vi "Q14070-Z030装调整机构.vi"() -> ()   [LabVIEW 2013]
panel:
  out "error out 3":errorcluster
  out "型号数量":i32=10
  out "KSJJ":string
  out "FGCS":string
  out "03RFID":string
  out "RFID读取完成":bool
  out "RFID读取触发":bool
  out "芯片ID":string
  out "产品ID":string
  in  "锁紧螺母批次号":string
  in  "调整螺塞批次号":string
  in  "弹簧批次号":string
  in  "O型圈批次号":string
  in  "支撑座批次号":string
  in  "复位按钮":bool
  in  "员工权限":bool
  in  "停止":bool
  in  "联线按钮":bool
  out "通讯状态":bool
  in  "选项卡控件 2":enum32{"自动", "手动", "参数查询"}(tab)
  out "本序完成":bool
  out "本序合格":bool
  out "上序完成":bool
  out "上序合格":bool
  out "取料操作状态":string
  out "取料工步号":dbl
  out "涂脂操作状态":string
  out "涂脂工步号":dbl
  out "流水线操作状态":string
  in  "流水线工步号":dbl
  out "报警提示":string
  out "报警工步号":dbl
  out "I上工位在位":bool
  out "I本工位在位":bool
  out "I下工位在位":bool
  out "I旋转气缸原位  2":bool
  out "I顶升气缸下位 2":bool
  out "I顶升气缸上位  2":bool
  out "I旋转气缸进位 2":bool
  out "I胶瓶在位":bool
  out "I辅具在位":bool
  out "I横孔涂脂在位":bool
  in  "M支撑座手动涂脂有效":bool
  in  "M图像识别涂脂开":bool
  in  "M图像识别触发":bool
  in  "M本工位放行":bool
  in  "M流水线旋转气缸原位":bool
  in  "M上工位放行":bool
  in  "M流水线顶升气缸下降":bool
  in  "M流水线旋转气缸旋转":bool
  in  "M横孔涂脂开":bool
  in  "M流水线顶升气缸顶升":bool
  out "I下工位在位":bool
  out "I上工位在位":bool
  out "I本工位在位":bool
  out "I旋转气缸进位":bool
  out "I顶升气缸上位":bool
  out "I顶升气缸下位":bool
  out "I旋转气缸原位":bool
  in  "参数修改":bool
  in  "参数查询":bool
  in  "参数列表":string[][](table)
  in  "员工ID":string
  out "员工姓名":string
  in  "型号选择":u16(ring)=1 items=["J706", "J709"]
  in  "参数加载":bool
  out "Q场景切换启动2":bool
  out "Q场景切换启动1":bool
  out "备用取料":i16=4
  out "error out 2":errorcluster
  out "ADODB._Connection Out":refnum<k7>
  out "error out":errorcluster
  out "Q场景切换 4":bool
  out "Q场景切换 3":bool
  out "Q场景切换 2":bool
  out "Q场景切换":bool
  out "场景切换选择":i16=4
  out "横孔涂脂设定次数":i16=4
  out "齿条支撑座涂脂设定次数":i16=4
  in  "M备用取料":bool
  out "产品选型":dbl
  # "芜湖机械转向器装配线"
  # "Z030 装调整机构"
  # "湖北唯思凌科装备制造有限公司 设计开发 (C)2015"
  # "Q14070机械转向器装配线"
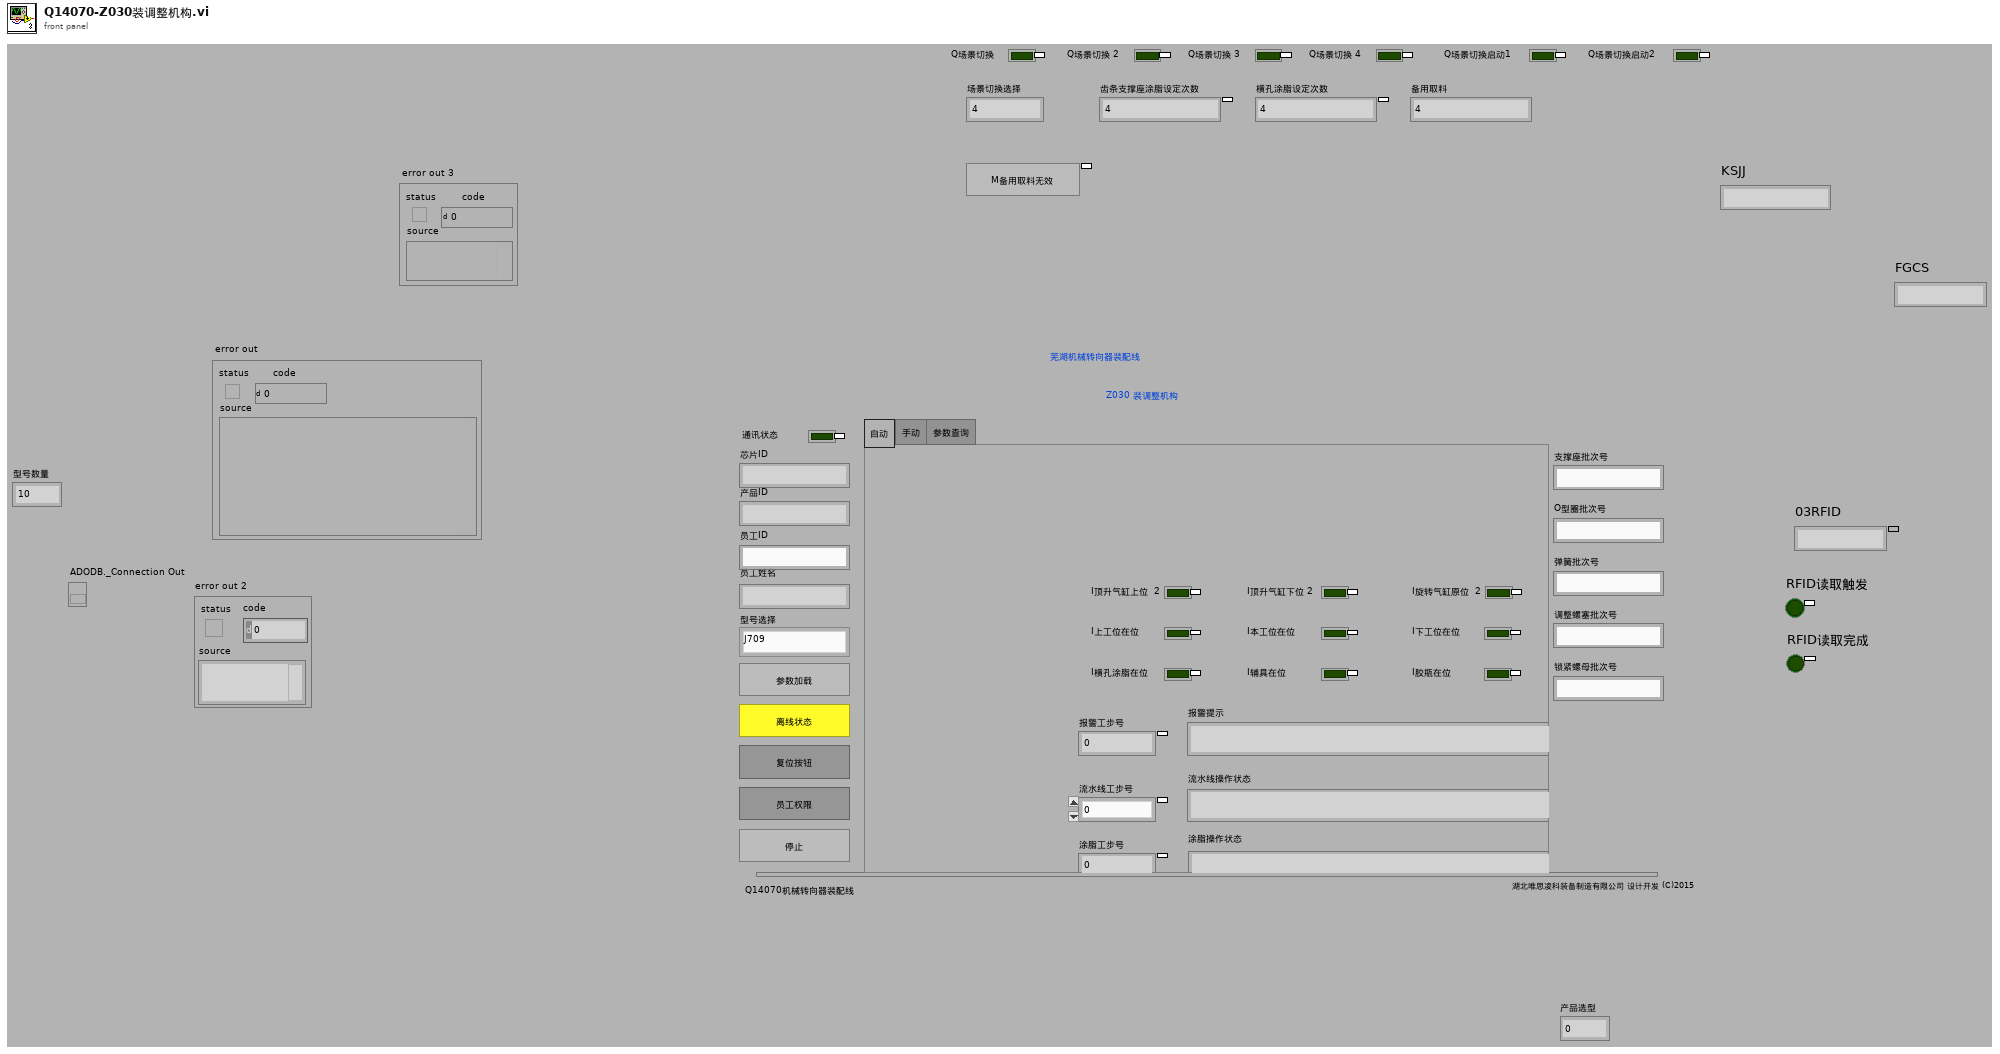
[diagram p1: front panel]
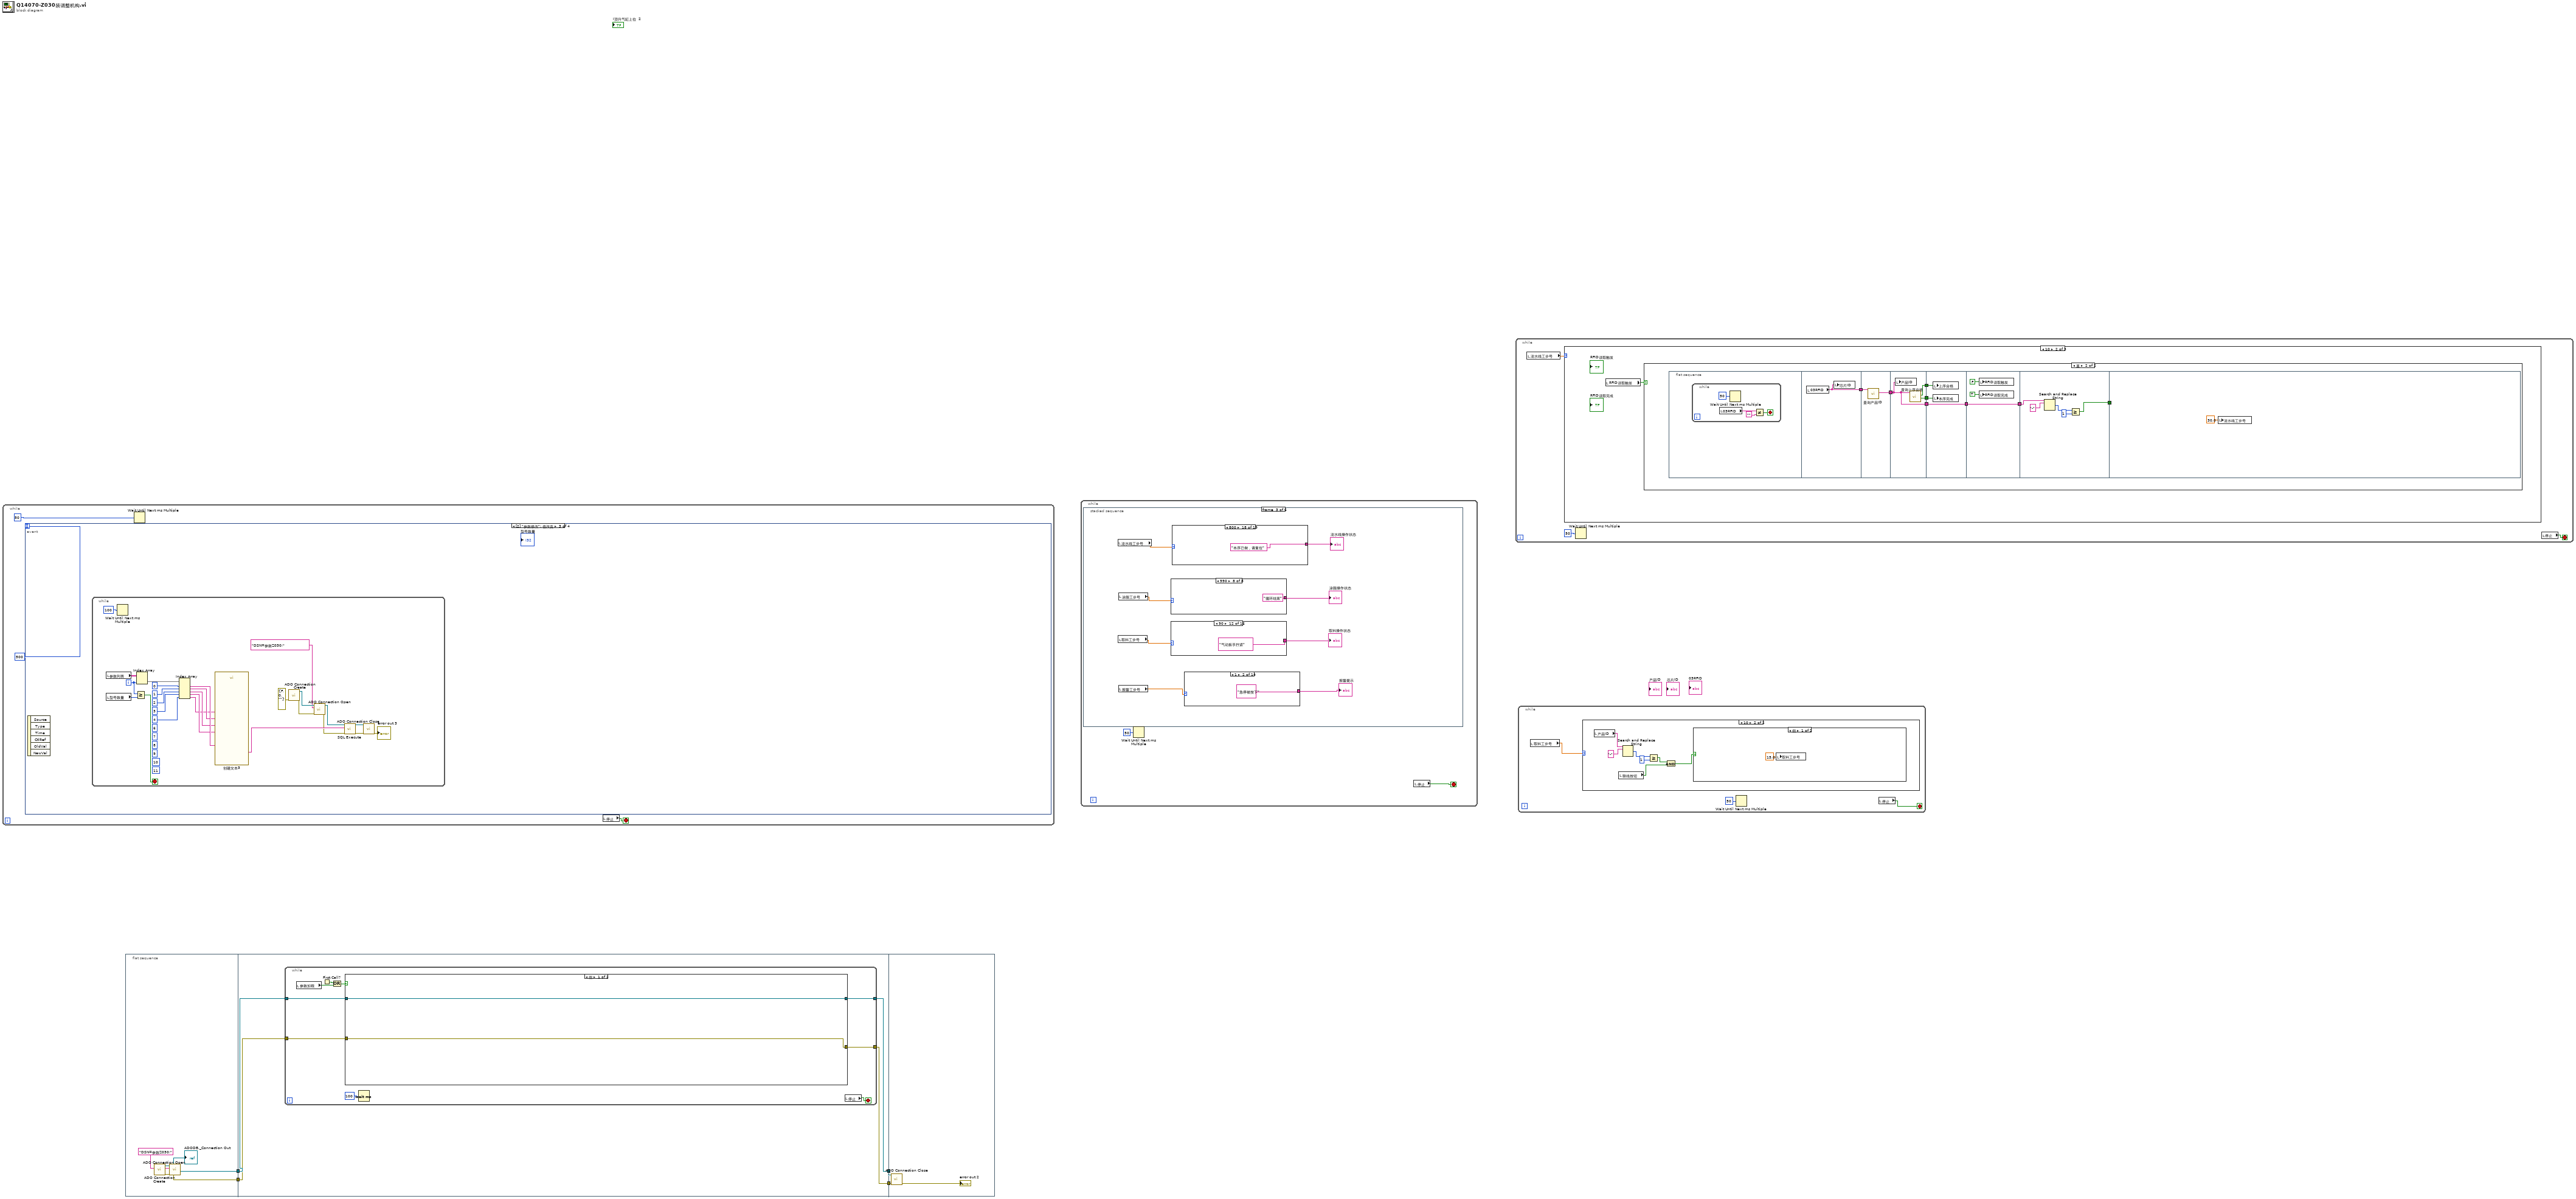
[diagram p0: block diagram]
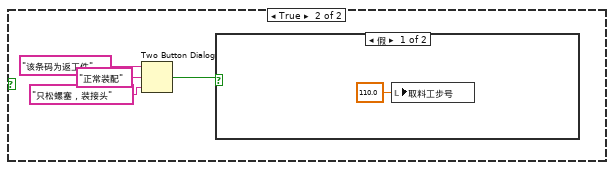
[diagram p3: hidden frame]
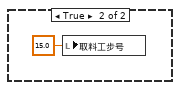
[diagram p4: hidden frame]
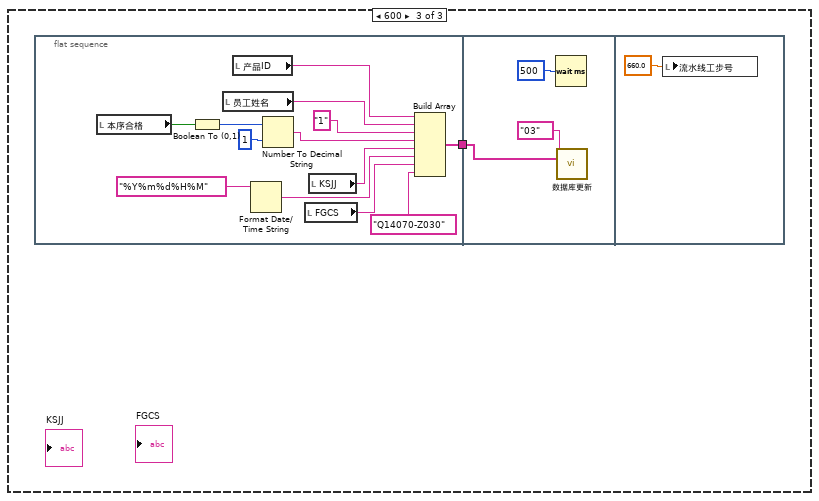
[diagram p7: hidden frame]
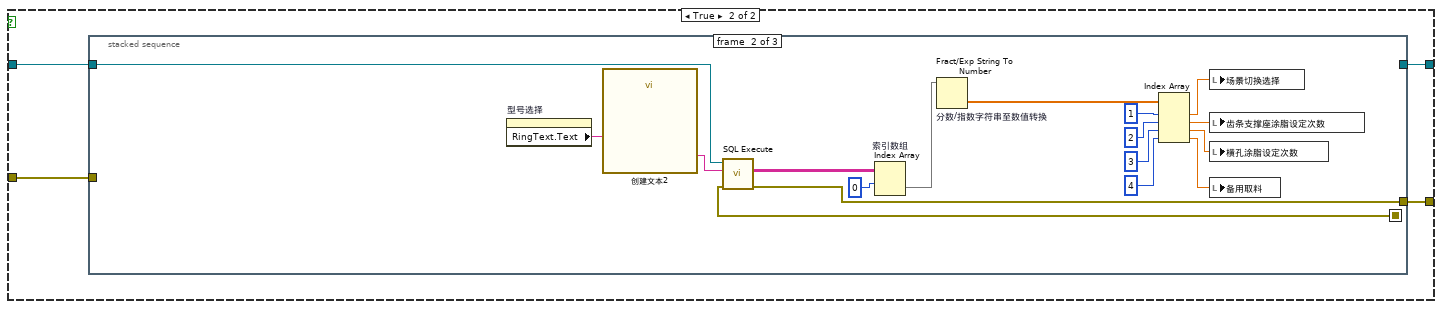
[diagram p8: hidden frame]
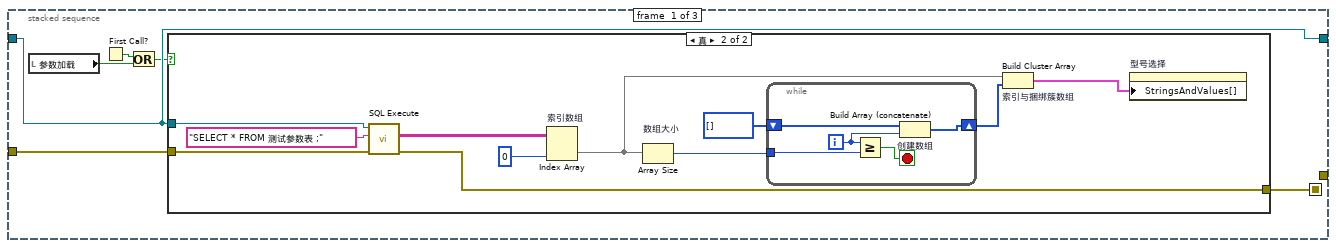
[diagram p9: hidden frame]
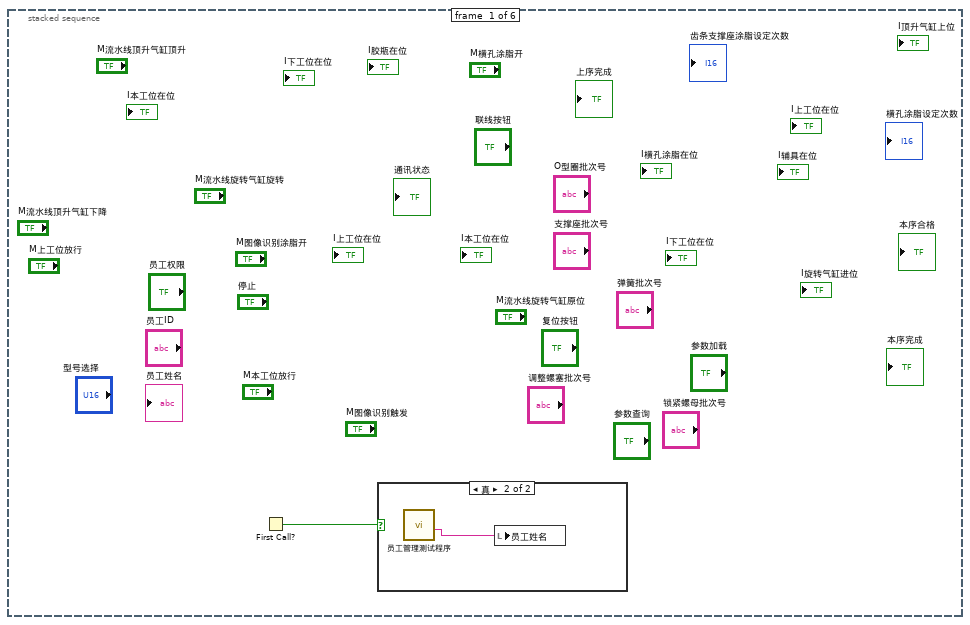
[diagram p12: hidden frame]
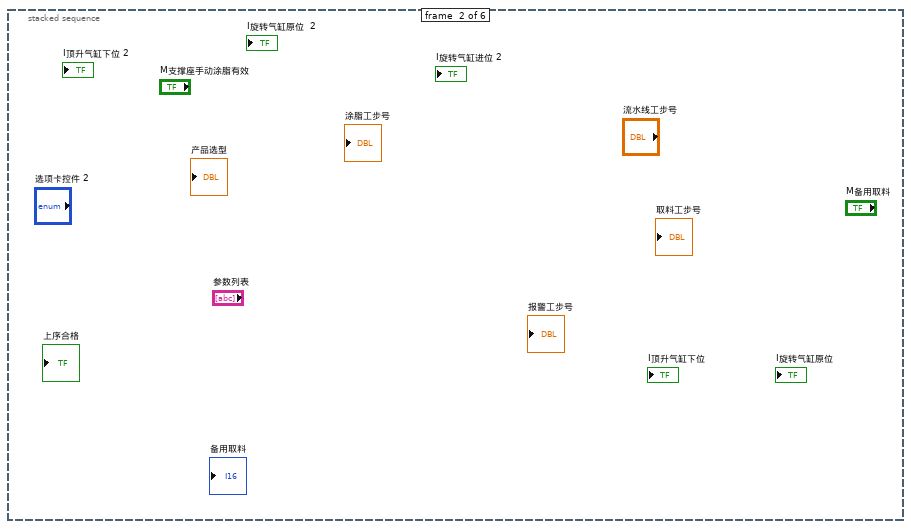
[diagram p14: hidden frame]
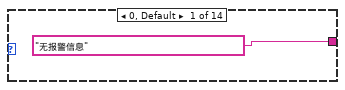
[diagram p15: hidden frame]
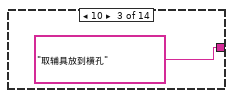
[diagram p16: hidden frame]
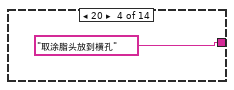
[diagram p17: hidden frame]
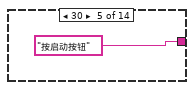
[diagram p18: hidden frame]
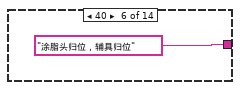
[diagram p19: hidden frame]
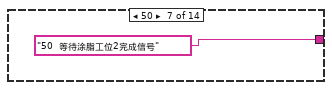
[diagram p20: hidden frame]
diagram:
  n1 = while {
    stop <- w5 stop-if-true
    n2 = event shown="[2] \"参数修改\": 值改变" {
      selector: _ -> [_ _ _ _]
      dyn-events: _ -> [_ _ _ _]
      timeout: 500 -> [_ _ _ _]
      event Timeout {
        n3 = event-data() -> ()  [unwired: 3 out]
      }
      event "参数查询": Value Change {
        n4 = event-data() -> ()  [unwired: 7 out]
        n5 = flat-sequence {
          tunnel: [w16] -> w13
          tunnel: [w26] -> w12
          tunnel: [w22] -> w11
          tunnel: [w19] -> w10
          tunnel: w13 -> [w31]
          tunnel: w12 -> [w29]
          tunnel: [w30] -> w9
          tunnel: w11 -> [w30]
          tunnel: [w29] -> w8
          tunnel: w10 -> [w28]
          tunnel: w9 -> [w34]
          tunnel: w8 -> [w33]
          frame #0 {
            n6 = call "字符串转换为数组.vi"("查询内容"=",产品型号,场景切换,图像识别位涂脂设定值,横孔涂脂设定值,备用取料有料") -> ("列首"=w14:string[])  [unwired: 10 in]
            n7 = property on="参数列表" class="Tbl (严格)"("Row Headers[]"=w14) -> ()  [unwired: 2 in, 2 out]
          }
          frame #1 {
            n8 = call "创建文本"() -> ("Result"=w27:string)  [unwired: 14 in, 1 out]
            n9 = call "ADO Connection Create.vi"() -> ("error out"=w21:errorcluster, "ADODB._Connection Out"=w25:refnum<k7>)  [unwired: 10 in]
            n10 = call "ADO Connection Open.vi"("error in (no error)"=w21, "ConnectionString"="DSN=参数Z030;", "ADODB._Connection In"=w25) -> ("error out"=w20:errorcluster, "ADODB._Connection Out"=w23:refnum<k7>)  [unwired: 7 in]
            n11 = call "SQL Execute.vi"("error in (no error)"=w20, "Command Text"=w27, "ADODB._Connection In"=w23) -> ("error out"=w26:errorcluster, "Data"=w18:string[][], "ADODB._Connection Out"=w22:refnum<k7>)  [unwired: 5 in, 1 out]
            n12 = Transpose 2D Array "二维数组转置"(2D array=w18) -> (transposed array=w16:string[][])
            n13 = Index Array(array=w16, index (row)=0 ("索引 (行)")) -> (element=w19:string[])  [unwired: 1 in]
          }
          frame #2 {
            n14 = local write "参数列表"(w31) -> ()
            n15 = property on="参数列表" class="Tbl (严格)"("Column Headers[]"=w28) -> ()  [unwired: 2 in, 2 out]
          }
          frame #3 {
            n16 = call "ADO Connection Close.vi"("error in (no error)"=w33, "ADODB._Connection In"=w34) -> ("error out"=→"error out":errorcluster)  [unwired: 8 in, 1 out]
          }
        }
      }
      event "参数修改": Value Change {
        n17 = event-data() -> ()  [unwired: 7 out]
        n18 = while {
          i -> [w57]
          stop <- w56 stop-if-true
          (unwired) 11 ("索引")
          (unwired) 10 ("索引")
          (unwired) 9 ("索引")
          (unwired) 8 ("索引")
          (unwired) 7 ("索引")
          (unwired) 6 ("索引")
          n19 = local read "参数列表"() -> (w59:string[][])
          n20 = local read "型号数量"() -> (w58:i32)
          n21 = Wait Until Next ms Multiple(millisecond multiple=u32 100 ("毫秒倍数")) -> ()  [unwired: 1 out]
          n22 = Greater Or Equal?(x=w57, y=w58) -> (x >= y?=w56:bool)
          n23 = Index Array(array=w59, index (col)=w57) -> (element=w51:string[])  [unwired: 1 in]
          n24 = Index Array(array=w51, index #1=0 ("索引"), index #2=1 ("索引"), index #3=2 ("索引"), index #4=3 ("索引"), index #5=4 ("索引")) -> (element #1=w46:string, element #2=w45:string, element #3=w44:string, element #4=w43:string, element #5=w42:string)
          n25 = call "创建文本3"("备用取料有料"=w42, "场景切换"=w45, "图像识别位涂脂设定值"=w44, "横孔涂脂设定值"=w43, "产品型号"=w46) -> ("Result"=w48:string)  [unwired: 9 in, 1 out]
          n26 = call "ADO Connection Create.vi"("error in (no error)"=errorcluster {"status"=FALSE, "code"=0, "source"=""}) -> ("error out"=w38:errorcluster, "ADODB._Connection Out"=w41:refnum<k7>)  [unwired: 9 in]
          n27 = call "ADO Connection Open.vi"("error in (no error)"=w38, "ConnectionString"="DSN=参数Z030;", "ADODB._Connection In"=w41) -> ("error out"=w39:errorcluster, "ADODB._Connection Out"=w40:refnum<k7>)  [unwired: 7 in]
          n28 = call "SQL Execute.vi"("error in (no error)"=w39, "Command Text"=w48, "ADODB._Connection In"=w40) -> ("error out"=w49:errorcluster, "ADODB._Connection Out"=w50:refnum<k7>)  [unwired: 5 in, 2 out]
          n29 = call "ADO Connection Close.vi"("error in (no error)"=w49, "ADODB._Connection In"=w50) -> ("error out"=→"error out 3":errorcluster)  [unwired: 8 in, 1 out]
        }
      }
      event "停止": Value Change {
        n30 = event-data() -> ()  [unwired: 7 out]
        n31 = flat-sequence {
          frame #0 {
            n32 = local write "涂脂工步号"(0.0 ("工步号")) -> ()
          }
          frame #1 {
            n33 = Wait Until Next ms Multiple(millisecond multiple=u32 1000 ("毫秒倍数")) -> ()  [unwired: 1 out]
          }
          frame #2 {
            n34 = Quit LabVIEW(quit? (T)=TRUE ("停止？(T)")) -> ()
          }
        }
      }
    }
    n35 = Wait Until Next ms Multiple(millisecond multiple=u32 50 ("毫秒倍数")) -> ()  [unwired: 1 out]
    n36 = local read "停止"() -> (w5:bool)
  }
  n37 = flat-sequence {
    tunnel: [w65] -> w4
    tunnel: [w64] -> w3
    tunnel: w4 -> [w72]
    tunnel: w3 -> [w71]
    tunnel: [w70] -> w2
    tunnel: [w69] -> w1
    tunnel: w2 -> [w129]
    tunnel: w1 -> [w128]
    frame #0 {
      n38 = call "ADO Connection Create.vi"() -> ("error out"=w67:errorcluster, "ADODB._Connection Out"=w68:refnum<k7>)  [unwired: 10 in]
      n39 = call "ADO Connection Open.vi"("error in (no error)"=w67, "ConnectionString"="DSN=参数Z030;", "ADODB._Connection In"=w68) -> ("error out"=w64:errorcluster, "ADODB._Connection Out"=w65:refnum<k7>)  [unwired: 7 in]
      "ADODB._Connection Out" <- w65
    }
    frame #1 {
      n40 = while {
        tunnel: w72 -> [w77]
        tunnel: w71 -> [w76]
        tunnel: [w75] -> w70
        tunnel: [w74] -> w69
        stop <- w80 stop-if-true
        n41 = local read "参数加载"() -> (w73:bool)
        n42 = First Call?() -> (First Call?: T/F=w79:bool)
        n43 = Or(x=w79, y=w73) -> (x .or. y?=w78:bool)
        n44 = case shown="假" w78 {
          tunnel: w77 -> [w83 w87]
          tunnel: w76 -> [w82 w86]
          tunnel: [w83 w85] -> w75
          tunnel: [w82 w84] -> w74
          frame False {
          }
          frame True {
            n45 = stacked-sequence {
              seq-local: [w91 _ _] -> [_ w125 _]
              tunnel: w87 -> [w92 w122 _]
              tunnel: w86 -> [w93 _ _]
              tunnel: [w92 _ _] -> w85
              tunnel: [_ w124 _] -> w84
              frame #0 {
                n46 = local read "参数加载"() -> (w89:bool)
                n47 = First Call?() -> (First Call?: T/F=w90:bool)
                n48 = Or(x=w90, y=w89) -> (x .or. y?=w88:bool)
                n49 = case shown="真" w88 {
                  tunnel: w93 -> [w94 w99]
                  tunnel: w92 -> [_ w97]
                  tunnel: [w94 w96] -> w91
                  frame False {
                  }
                  frame True {
                    n50 = call "SQL Execute.vi"("error in (no error)"=w99, "Command Text"="SELECT * FROM 测试参数表 ;", "ADODB._Connection In"=w97) -> ("error out"=w96:errorcluster, "Data"=w100:string[][])  [unwired: 5 in, 2 out]
                    n51 = Index Array "索引数组"(array=w100, index (col)=0 ("禁用的索引 (列)")) -> (element=w103:string[])  [unwired: 1 in]
                    n52 = Array Size "数组大小"(array=w103) -> (size(s)=w102:i32)
                    n53 = while {
                      shift-right: [w108] -> w101
                      shift-left: i32[] [] -> [w109]
                      tunnel: w102 -> [w106]
                      i -> [w107]
                      stop <- w110 stop-if-true
                      n54 = Greater Or Equal?(x=w107, y=w106) -> (x >= y?=w110:bool)
                      n55 = Build Array (concatenate) "创建数组"(w109, w107) -> (w108:i32[])
                    }
                    n56 = Build Cluster Array "索引与捆绑簇数组"(w103, w101) -> (w95:cluster{"String":string, i32}[])
                    n57 = property on="型号选择" class="Ring (严格)"("StringsAndValues[]"=w95) -> ()  [unwired: 2 in, 2 out]
                  }
                }
              }
              frame #1 {
                n58 = property on="型号选择" class="Ring (严格)"() -> ("RingText.Text"=w121:string)  [unwired: 2 in, 2 out]
                n59 = call "创建文本2"("产品型号"=w121) -> ("Result"=w123:string)  [unwired: 13 in, 1 out]
                n60 = call "SQL Execute.vi"("error in (no error)"=w125, "Command Text"=w123, "ADODB._Connection In"=w122) -> ("error out"=w124:errorcluster, "Data"=w127:string[][])  [unwired: 5 in, 2 out]
                n61 = Index Array "索引数组"(array=w127, index (row)=0 ("索引 (行)")) -> (element=w120:string[])  [unwired: 1 in]
                n62 = Fract/Exp String To Number "分数/指数字符串至数值转换"(string=w120) -> (number=w115:dbl[])  [unwired: 3 in, 1 out]
                n63 = Index Array(array=w115, index #1=1 ("索引"), index #2=2 ("索引"), index #3=3 ("索引"), index #4=4 ("索引")) -> (element #1=w114:dbl, element #2=w113:dbl, element #3=w112:dbl, element #4=w111:dbl)
                n64 = local write "场景切换选择"(w114) -> ()
                n65 = local write "齿条支撑座涂脂设定次数"(w113) -> ()
                n66 = local write "横孔涂脂设定次数"(w112) -> ()
                n67 = local write "备用取料"(w111) -> ()
              }
              frame #2 {
              }
            }
          }
        }
        n68 = Wait (ms)(milliseconds to wait=u32 100 ("等待时间（毫秒）")) -> ()  [unwired: 1 out]
        n69 = local read "停止"() -> (w80:bool)
      }
    }
    frame #2 {
      n70 = call "ADO Connection Close.vi"("error in (no error)"=w128, "ADODB._Connection In"=w129) -> ("error out"=→"error out 2":errorcluster)  [unwired: 8 in, 1 out]
    }
  }
  n71 = while {
    stop <- w131 stop-if-true
    n72 = stacked-sequence {
      frame #0 {
        n73 = First Call?() -> (First Call?: T/F=w133:bool)
        n74 = case shown="真" w133 {
          frame False {
          }
          frame True {
            n75 = call "员工管理测试程序.vi"() -> ("员工姓名"=w134:string)  [unwired: 11 in]
            n76 = local write "员工姓名"(w134) -> ()
          }
        }
      }
      frame #1 {
      }
      frame #2 {
        n77 = local read "流水线工步号"() -> (w142:dbl)
        n78 = local read "取料工步号"() -> (w138:dbl)
        n79 = local read "涂脂工步号"() -> (w139:dbl)
        n80 = local read "报警工步号"() -> (w136:dbl)
        n81 = case shown="90" w138 {
          tunnel: ["等待流水线准备好" ("工步操作状态") "取辅具放到横孔" ("工步操作状态") "取涂脂头放到横孔" ("工步操作状态") "按横孔涂脂按钮" ("工步操作状态") "涂脂头归位，辅具归位" ("工步操作状态") "  等待支撑座涂脂完成信号" ("工步操作状态") " 取调整螺塞" ("工步操作状态") " 取调整螺塞胶" ("工步操作状态") "放回调整螺塞胶" ("工步操作状态") "80 取弹簧" ("工步操作状态") "" ("工步操作状态") "气动扳手拧紧" ("工步操作状态") "100 取锁紧螺母" ("工步操作状态") " 定扭扳手定扭" ("工步操作状态") "120 取料完成" ("工步操作状态") "循环结束" ("工步操作状态")] -> w137
          frame 0, Default {
          }
          frame 10 {
          }
          frame 20 {
          }
          frame 30 {
          }
          frame 40 {
          }
          frame 50 {
          }
          frame 70 {
          }
          frame 75 {
          }
          frame 77 {
          }
          frame 80 {
          }
          frame 85 {
          }
          frame 90 {
          }
          frame 100 {
          }
          frame 110 {
          }
          frame 120 {
          }
          frame 990 {
          }
        }
        "取料操作状态" <- w137
        n82 = case shown="990" w139 {
          tunnel: ["等待涂脂启动" ("工步操作状态") "10 取齿条支撑座总成" ("工步操作状态") "20 取O型圈" ("工步操作状态") "25 按涂脂按钮" ("工步操作状态") "30 检测工件有无" ("工步操作状态") " 手动下按支撑座涂脂按钮" ("工步操作状态") "40  自动涂脂" ("工步操作状态") "循环结束" ("工步操作状态")] -> w140
          frame 0, Default {
          }
          frame 10 {
          }
          frame 20 {
          }
          frame 25 {
          }
          frame 30 {
          }
          frame 35 {
          }
          frame 40 {
          }
          frame 990 {
          }
        }
        "涂脂操作状态" <- w140
        n83 = case shown="800" w142 {
          tunnel: ["等待启动" ("工步操作状态") "RFID读取触发" ("工步操作状态") "" ("工步操作状态") "上序合格判断" ("工步操作状态") "" ("工步操作状态") "上阻挡器放行" ("工步操作状态") "本工位在位检测" ("工步操作状态") "流水线顶升" ("工步操作状态") "流水线夹具旋转" ("工步操作状态") "流水线准备好,等待取料完成信号" ("工步操作状态") "等待取料完成" ("工步操作状态") "给出本工位合格和完成信号" ("工步操作状态") "按下放行按钮后，夹具旋转" ("工步操作状态") "流水线顶升气缸下降" ("工步操作状态") "本工位放行" ("工步操作状态") "本工位放行完成" ("工步操作状态") "数据上传完成" ("工步操作状态") "本序已做，请复位" ("工步操作状态") "循环结束" ("工步操作状态")] -> w141
          frame 0, Default {
          }
          frame 10 {
          }
          frame 20 {
          }
          frame 30 {
          }
          frame 40 {
          }
          frame 70 {
          }
          frame 80 {
          }
          frame 95 {
          }
          frame 100 {
          }
          frame 200 {
          }
          frame 500 {
          }
          frame 520 {
          }
          frame 540 {
          }
          frame 550 {
          }
          frame 560 {
          }
          frame 580 {
          }
          frame 660 {
          }
          frame 800 {
          }
          frame 990 {
          }
        }
        "流水线操作状态" <- w141
        n84 = case shown="1" w136 {
          tunnel: ["无报警信息" ("工步操作状态") "急停被按下" ("工步操作状态") "取辅具放到横孔" ("工步操作状态") "取涂脂头放到横孔" ("工步操作状态") "按启动按钮" ("工步操作状态") "涂脂头归位，辅具归位" ("工步操作状态") "50  等待涂脂工位2完成信号" ("工步操作状态") " 取弹簧" ("工步操作状态") "80 取调整螺塞" ("工步操作状态") "90 气动扳手拧紧" ("工步操作状态") "100 取锁紧螺母" ("工步操作状态") "110 定扭扳手定扭" ("工步操作状态") "120 取料完成" ("工步操作状态") "循环结束" ("工步操作状态")] -> w135
          frame 0, Default {
          }
          frame 1 {
          }
          frame 10 {
          }
          frame 20 {
          }
          frame 30 {
          }
          frame 40 {
          }
          frame 50 {
          }
          frame 70 {
          }
          frame 80 {
          }
          frame 90 {
          }
          frame 100 {
          }
          frame 110 {
          }
          frame 120 {
          }
          frame 990 {
          }
        }
        "报警提示" <- w135
      }
      frame #3 {
        n85 = local read "场景切换选择"() -> (w200:i16)
        n86 = case shown="0" w200 {
          frame 0 {
            w201 = FALSE
            n87 = local write "Q场景切换"(w201) -> ()
            n88 = local write "Q场景切换 4"(w201) -> ()
            n89 = local write "Q场景切换 2"(w201) -> ()
            n90 = local write "Q场景切换 3"(w201) -> ()
          }
          frame 1 {
            w203 = FALSE
            n91 = local write "Q场景切换"(TRUE ("Q场景切换")) -> ()
            n92 = local write "Q场景切换 4"(w203) -> ()
            n93 = local write "Q场景切换 2"(w203) -> ()
            n94 = local write "Q场景切换 3"(w203) -> ()
          }
          frame 2 {
            w204 = FALSE
            n95 = local write "Q场景切换"(w204) -> ()
            n96 = local write "Q场景切换 4"(w204) -> ()
            n97 = local write "Q场景切换 2"(TRUE ("Q场景切换")) -> ()
            n98 = local write "Q场景切换 3"(w204) -> ()
          }
          frame 3 {
            w207 = TRUE ("Q场景切换")
            w206 = FALSE
            n99 = local write "Q场景切换"(w207) -> ()
            n100 = local write "Q场景切换 4"(w206) -> ()
            n101 = local write "Q场景切换 2"(w207) -> ()
            n102 = local write "Q场景切换 3"(w206) -> ()
          }
          frame 4 {
            w208 = FALSE
            n103 = local write "Q场景切换"(w208) -> ()
            n104 = local write "Q场景切换 4"(w208) -> ()
            n105 = local write "Q场景切换 2"(w208) -> ()
            n106 = local write "Q场景切换 3"(TRUE ("Q场景切换")) -> ()
          }
          frame 5 {
            w211 = TRUE ("Q场景切换")
            w210 = FALSE
            n107 = local write "Q场景切换"(w211) -> ()
            n108 = local write "Q场景切换 4"(w210) -> ()
            n109 = local write "Q场景切换 2"(w210) -> ()
            n110 = local write "Q场景切换 3"(w211) -> ()
          }
          frame 6 {
            w213 = TRUE ("Q场景切换")
            w212 = FALSE
            n111 = local write "Q场景切换"(w212) -> ()
            n112 = local write "Q场景切换 4"(w212) -> ()
            n113 = local write "Q场景切换 2"(w213) -> ()
            n114 = local write "Q场景切换 3"(w213) -> ()
          }
          frame 7 {
            w215 = TRUE ("Q场景切换")
            n115 = local write "Q场景切换"(w215) -> ()
            n116 = local write "Q场景切换 4"(FALSE) -> ()
            n117 = local write "Q场景切换 2"(w215) -> ()
            n118 = local write "Q场景切换 3"(w215) -> ()
          }
          frame 8 {
            w216 = FALSE
            n119 = local write "Q场景切换"(w216) -> ()
            n120 = local write "Q场景切换 4"(TRUE ("Q场景切换")) -> ()
            n121 = local write "Q场景切换 2"(w216) -> ()
            n122 = local write "Q场景切换 3"(w216) -> ()
          }
          frame 32, Default {
          }
        }
      }
      frame #4 {
        n123 = local read "备用取料"() -> (w218:i16)
        n124 = case shown="1" w218 {
          frame 0 {
            n125 = local write "M备用取料"(FALSE ("M备用取料")) -> ()
          }
          frame 1 {
            n126 = local write "M备用取料"(TRUE ("M备用取料")) -> ()
          }
          frame 2, Default {
          }
        }
      }
      frame #5 {
        n127 = local read "参数加载"() -> (w221:bool)
        n128 = case shown="真" w221 {
          frame False {
          }
          frame True {
            n129 = flat-sequence {
              frame #0 {
                n130 = Wait Until Next ms Multiple(millisecond multiple=u32 1000 ("毫秒计时值")) -> ()  [unwired: 1 out]
              }
              frame #1 {
                w223 = TRUE
                "Q场景切换启动2" <- w223
                "Q场景切换启动1" <- w223
              }
              frame #2 {
                n131 = Wait Until Next ms Multiple(millisecond multiple=u32 1000 ("毫秒计时值")) -> ()  [unwired: 1 out]
              }
              frame #3 {
                w225 = FALSE
                n132 = local write "Q场景切换启动1"(w225) -> ()
                n133 = local write "Q场景切换启动2"(w225) -> ()
              }
            }
          }
        }
      }
    }
    n134 = Wait Until Next ms Multiple(millisecond multiple=u32 50 ("毫秒倍数")) -> ()  [unwired: 1 out]
    n135 = local read "停止"() -> (w131:bool)
  }
  n136 = while {
    stop <- w227 stop-if-true
    n137 = local read "流水线工步号"() -> (w226:dbl)
    n138 = case shown="10" w226 {
      frame 0, Default {
      }
      frame 10 {
        n139 = local read "RFID读取触发"() -> (w229:bool)
        n140 = case shown="真" w229 {
          frame False {
          }
          frame True {
            n141 = flat-sequence {
              tunnel: [w242] -> w237
              tunnel: w237 -> [w244]
              tunnel: [w243] -> w236
              tunnel: w236 -> [w245]
              tunnel: [w247] -> w235
              tunnel: [w246] -> w234
              tunnel: [w245] -> w233
              tunnel: w235 -> [w250]
              tunnel: w234 -> [w249]
              tunnel: w233 -> [w248]
              tunnel: [w248] -> w232
              tunnel: w232 -> [w251]
              tunnel: [w251] -> w231
              tunnel: w231 -> [w258]
              tunnel: [w254] -> w230
              tunnel: w230 -> [_]
              frame #0 {
                n142 = while {
                  stop <- w239 stop-if-true
                  n143 = local read "03RFID"() -> (w241:string)
                  n144 = Wait Until Next ms Multiple(millisecond multiple=u32 50 ("毫秒倍数")) -> ()  [unwired: 1 out]
                  n145 = Not Equal?(x=w241, y="") -> (x != y?=w239:bool)
                }
              }
              frame #1 {
                n146 = local read "03RFID"() -> (w242:string)
                n147 = local write "芯片ID"(w242) -> ()
              }
              frame #2 {
                n148 = call "查询产品ID.vi"("芯片编码"=w244) -> ("产品ID"=w243:string)  [unwired: 8 in, 2 out]
              }
              frame #3 {
                n149 = local write "产品ID"(w245) -> ()
                n150 = call "查询上序合格.vi"("产品ID"=w245) -> ("本序已做"=w246:bool, "上序合格"=w247:bool)  [unwired: 8 in, 1 out]
              }
              frame #4 {
                n151 = local write "上序合格"(w250) -> ()
                n152 = local write "本序完成"(w249) -> ()
              }
              frame #5 {
                n153 = local write "RFID读取触发"(FALSE ("RFID读取触发")) -> ()
                n154 = local write "RFID读取完成"(TRUE ("RFID读取完成")) -> ()
              }
              frame #6 {
                n155 = Search and Replace String(input string=w258, search string="-" ("搜索字符串")) -> (number of replacements=w256:i32)  [unwired: 6 in, 3 out]
                n156 = Greater Or Equal?(x=w256, y=1) -> (x >= y?=w254:bool)
              }
              frame #7 {
                n157 = local write "流水线工步号"(30.0 ("工步号")) -> ()
              }
            }
          }
        }
      }
      frame 600 {
        n158 = flat-sequence {
          tunnel: [w264] -> w260
          tunnel: w260 -> [w274]
          frame #0 {
            n159 = local read "本序合格"() -> (w269:bool)
            n160 = Boolean To (0,1)(Boolean=w269) -> (0, 1=w273:i16)
            n161 = local read "员工姓名"() -> (w270:string)
            n162 = local read "产品ID"() -> (w263:string)
            n163 = Format Date/Time String(time format string (%c)="%Y%m%d%H%M" ("时间格式字符串(%c)")) -> (date/time string=w271:string)  [unwired: 2 in]
            n164 = Number To Decimal String(number=w273, width (-)=i16 1 ("宽度(-)")) -> (decimal integer string=w261:string)
            n165 = local read "FGCS"() -> (w266:string)
            n166 = local read "KSJJ"() -> (w268:string)
            n167 = Build Array(w263, w270, "1" ("元素"), w261, w268, w271, w266, "Q14070-Z030") -> (w264:string[])
          }
          frame #1 {
            n168 = Wait (ms)(milliseconds to wait=u32 500 ("等待时间（毫秒）")) -> ()  [unwired: 1 out]
            n169 = call "数据库更新.vi"("设备号"="03", "数据"=w274) -> ()  [unwired: 13 in, 1 out]
          }
          frame #2 {
            n170 = local write "流水线工步号"(660.0 ("工步号")) -> ()
          }
        }
      }
    }
    n171 = Wait Until Next ms Multiple(millisecond multiple=u32 50 ("毫秒倍数")) -> ()  [unwired: 1 out]
    n172 = local read "停止"() -> (w227:bool)
  }
  n173 = while {
    stop <- w279 stop-if-true
    n174 = local read "取料工步号"() -> (w278:dbl)
    n175 = case shown="10" w278 {
      frame 0, Default {
      }
      frame 10 {
        n176 = local read "产品ID"() -> (w284:string)
        n177 = local read "联线按钮"() -> (w282:bool)
        n178 = Search and Replace String(input string=w284, search string="-" ("搜索字符串")) -> (number of replacements=w286:i32)  [unwired: 6 in, 3 out]
        n179 = Greater Or Equal?(x=w286, y=1) -> (x >= y?=w283:bool)
        n180 = And(x=w283, y=w282) -> (x .and. y?=w281:bool)
        n181 = case shown="假" w281 {
          frame False {
            n182 = local write "取料工步号"(15.0 ("取料工步号")) -> ()
          }
          frame True {
            n183 = Two Button Dialog(message="该条码为返工件" ("消息"), 1:"只松螺塞，装接头" ("F按钮名称（“取消”）"), 2:"正常装配" ("T按钮名称（“确定”）")) -> (T button?=w289:bool)
            n184 = case shown="假" w289 {
              frame False {
                n185 = local write "取料工步号"(110.0 ("取料工步号")) -> ()
              }
              frame True {
                n186 = local write "取料工步号"(15.0 ("取料工步号")) -> ()
              }
            }
          }
        }
      }
    }
    n187 = Wait Until Next ms Multiple(millisecond multiple=u32 50 ("毫秒倍数")) -> ()  [unwired: 1 out]
    n188 = local read "停止"() -> (w279:bool)
  }
